vi "CmdConsole.Kill.vi"(8 "error in":errorcluster, 11 "CmdConsole in":refnum<class "CmdConsole.lvclass">) -> (0 "error out":errorcluster, 3 "CmdConsole out":refnum<class "CmdConsole.lvclass">)   [LabVIEW 2024, in "CmdConsole.lvclass"]
uses:
  CmdConsole.lvclass
  CmdConsole.lvclass/CmdConsole.ctl
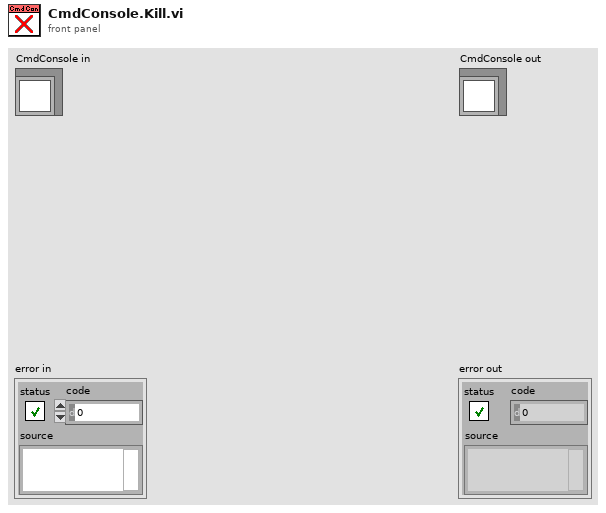
[diagram p1: front panel]
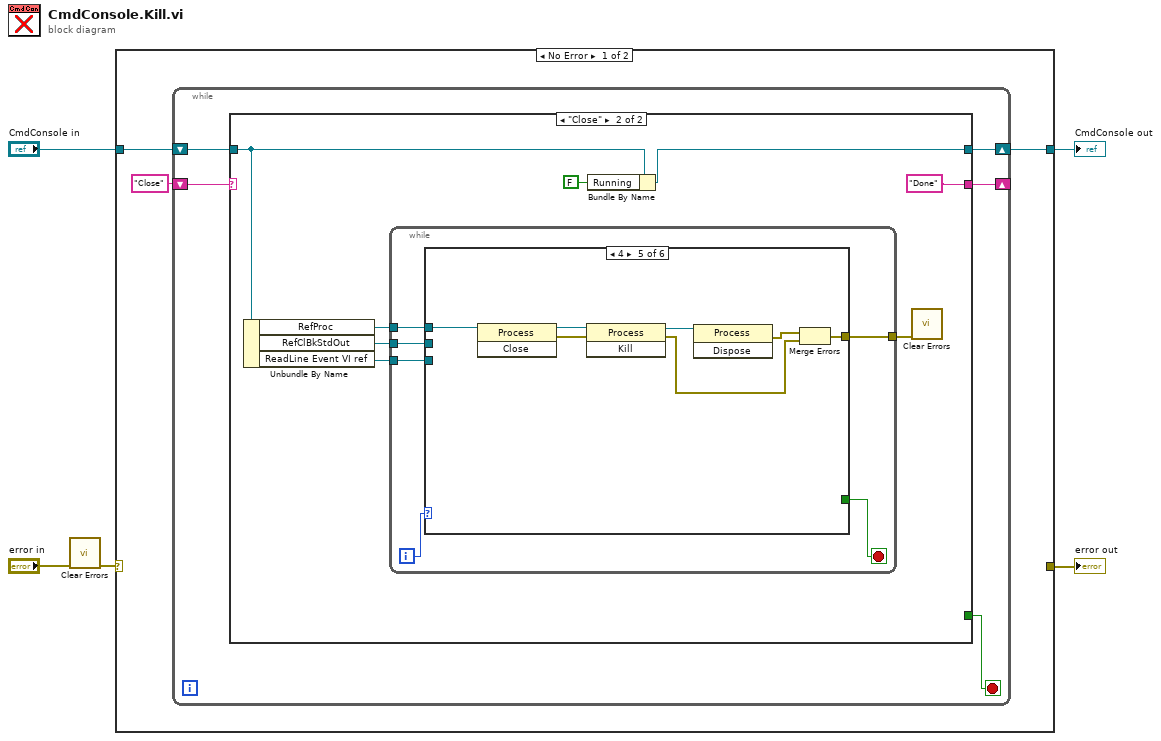
[diagram p0: block diagram]
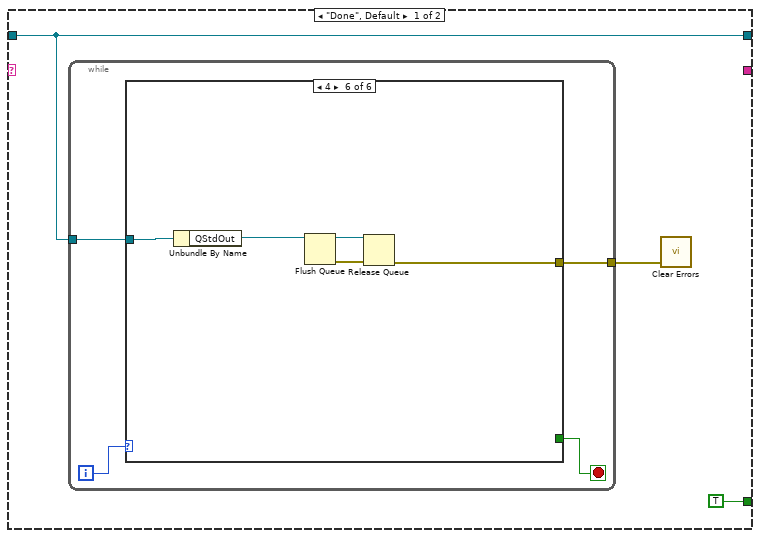
[diagram p2: hidden frame]
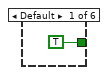
[diagram p3: hidden frame]
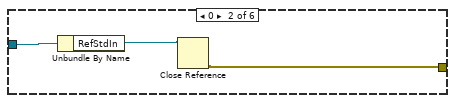
[diagram p4: hidden frame]
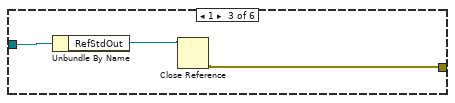
[diagram p5: hidden frame]
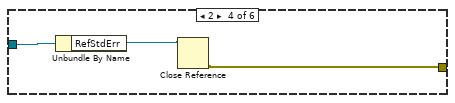
[diagram p6: hidden frame]
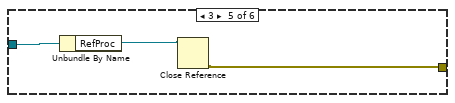
[diagram p7: hidden frame]
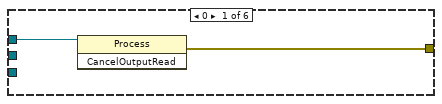
[diagram p8: hidden frame]
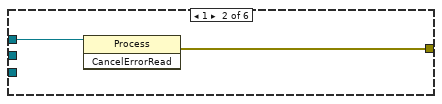
[diagram p9: hidden frame]
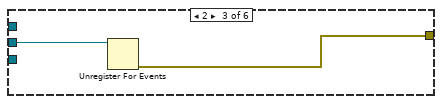
[diagram p10: hidden frame]
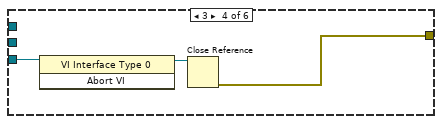
[diagram p11: hidden frame]
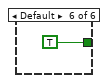
[diagram p12: hidden frame]
diagram:
  n1 = call <vilib>:"Clear Errors.vi"("error in (no error)"="error in") -> ("error out"=w2:errorcluster)  [unwired: 5 in, 1 out]
  n2 = case shown="No Error" w2 {
    selector: w2 -> [_ w71]
    tunnel: [_ w71] -> w5
    tunnel: [w7 w70] -> w3
    tunnel: "CmdConsole in" -> [w8 w70]
    frame No Error {
      n3 = while {
        shift-right: [w12] -> w7
        shift-left: w8 -> [w11]
        shift-right: [w13] -> _
        shift-left: "Close" -> [w10]
        stop <- w9 stop-if-true
        n4 = case shown="\"Close\"" w10 {
          tunnel: w11 -> [w15 w45]
          tunnel: [_ "Done"] -> w13
          tunnel: [w15 w44] -> w12
          tunnel: [TRUE _] -> w9
          frame "Done", Default {
            n5 = while {
              tunnel: w15 -> [w20]
              tunnel: [w17] -> w14
              i -> [w19]
              stop <- w18 stop-if-true
              n6 = case shown="4" w19 {
                tunnel: w20 -> [_ w24 w27 w30 w33 w38]
                tunnel: [TRUE _ _ _ _ _] -> w18
                tunnel: [_ w22 w25 w28 w31 w37] -> w17
                frame Default {
                }
                frame 0 {
                  n7 = Unbundle By Name(w24) -> ("RefStdIn"=w23:refnum<k24>)
                  n8 = Close Reference(reference=w23) -> (error out=w22:errorcluster)  [unwired: 1 in]
                }
                frame 1 {
                  n9 = Unbundle By Name(w27) -> ("RefStdOut"=w26:refnum<k24>)
                  n10 = Close Reference(reference=w26) -> (error out=w25:errorcluster)  [unwired: 1 in]
                }
                frame 2 {
                  n11 = Unbundle By Name(w30) -> ("RefStdErr"=w29:refnum<k24>)
                  n12 = Close Reference(reference=w29) -> (error out=w28:errorcluster)  [unwired: 1 in]
                }
                frame 3 {
                  n13 = Unbundle By Name(w33) -> ("RefProc"=w32:refnum<k24>)
                  n14 = Close Reference(reference=w32) -> (error out=w31:errorcluster)  [unwired: 1 in]
                }
                frame 4 {
                  n15 = Unbundle By Name(w38) -> ("QStdOut"=w34:refnum<queue>)
                  n16 = Flush Queue(queue=w34) -> (queue out=w36:refnum<queue>, error out=w35:errorcluster)  [unwired: 1 in, 1 out]
                  n17 = Release Queue(queue=w36, error in (no error)=w35) -> (error out=w37:errorcluster)  [unwired: 1 in, 2 out]
                }
              }
            }
            n18 = call <vilib>:"Clear Errors.vi"("error in (no error)"=w14) -> ()  [unwired: 5 in, 2 out]
          }
          frame "Close" {
            n19 = Unbundle By Name(w45) -> ("RefProc"=w42:refnum<k24>, "RefClBkStdOut"=w41:refnum<k27>, "ReadLine Event VI ref"=w40:refnum<vi>)
            n20 = while {
              tunnel: w42 -> [w51]
              tunnel: w41 -> [w49]
              tunnel: w40 -> [w48]
              tunnel: [w47] -> w39
              i -> [w52]
              stop <- w50 stop-if-true
              n21 = case shown="4" w52 {
                tunnel: w51 -> [w54 w56 _ _ w68 _]
                tunnel: [_ _ _ _ _ TRUE] -> w50
                tunnel: [w53 w55 w57 w59 w65 _] -> w47
                tunnel: w49 -> [_ _ w58 _ _ _]
                tunnel: w48 -> [_ _ _ w60 _ _]
                frame 0 {
                  n22 = invoke class="Process" method="CancelOutputRead"(reference=w54) -> (error out=w53:errorcluster)  [unwired: 2 in, 2 out]
                }
                frame 1 {
                  n23 = invoke class="Process" method="CancelErrorRead"(reference=w56) -> (error out=w55:errorcluster)  [unwired: 2 in, 2 out]
                }
                frame 2 {
                  n24 = Unregister For Events(event registration refnum=w58) -> (error out=w57:errorcluster)  [unwired: 1 in]
                }
                frame 3 {
                  n25 = invoke class="VI Interface Type 0" method="Abort VI"(reference=w60) -> (reference out=w61:refnum<vi>)  [unwired: 2 in, 2 out]
                  n26 = Close Reference(reference=w61) -> (error out=w59:errorcluster)  [unwired: 1 in]
                }
                frame 4 {
                  n27 = invoke class="Process" method="Close"(reference=w68) -> (reference out=w67:refnum<k24>, error out=w64:errorcluster)  [unwired: 2 in, 1 out]
                  n28 = invoke class="Process" method="Kill"(reference=w67, error in=w64) -> (reference out=w66:refnum<k24>, error out=w63:errorcluster)  [unwired: 1 in, 1 out]
                  n29 = invoke class="Process" method="Dispose"(reference=w66) -> (error out=w62:errorcluster)  [unwired: 2 in, 2 out]
                  n30 = Merge Errors(w62, w63) -> (w65:errorcluster)
                }
                frame Default {
                }
              }
            }
            n31 = Bundle By Name(cluster=w45, "Running"=FALSE) -> (w44:refnum<class "CmdConsole.lvclass">)
            n32 = call <vilib>:"Clear Errors.vi"("error in (no error)"=w39) -> ()  [unwired: 5 in, 2 out]
          }
        }
      }
    }
    frame Error {
    }
  }
  "error out" <- w5
  "CmdConsole out" <- w3
